vi "initialize Session Data.vi"(0 "OBJ - Session in":refnum<class "FPGA Session.lvclass">, 11 "error in":errorcluster) -> (4 "OBJ - Session out":refnum<class "FPGA Session.lvclass">, 15 "error out":errorcluster)   [LabVIEW 2015, in "FPGA Session.lvclass"]
doc: "OVERRIDE VI\nPlaceholder for decendant sessions to initialize and set their default values"
uses:
  FPGA Session.lvclass
  FPGA Session.lvclass/FPGA Session.ctl
  <vilib>/Utility/error.llb/Error Cluster From Error Code.vi
  <vilib>/rvi/errors/niLvFpgaAdjustHostInterfaceError.vi
  <vilib>/RVI Host/nirviSupport.llb/nirviErrorClusterFromErrorCode.vi
  <vilib>/FPGAPlugInAG/cRIO-9081/niLvFpga_Open_cRIO-9081.vi
  FPGA Ref.ctl
  <vilib>/rvi/interface/nirviMethod/nirviMethod.xnode
  FPGA Bitfiles/NickIO.lvbitx
  <vilib>/rvi/interface/nirviOpenFPGA/nirviOpenFPGA.xnode
  <vilib>/rvi/interface/nirviMethod/StockFPGA_InlinedMethodWaitForSingleIRQ.vi
  <vilib>/FPGAPlugInAG/cRIO-9081/niLvFpga_WaitOnIrq_cRIO-9081.vi
  <vilib>/FPGAPlugInAG/cRIO-9081/niLvFpga_AcknowledgeIrq_cRIO-9081.vi
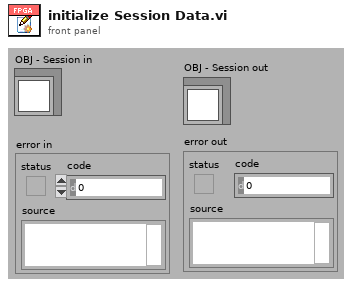
[diagram p1: front panel]
types:
  T1 = typedef "FPGA Ref.ctl" = refnum<k20>
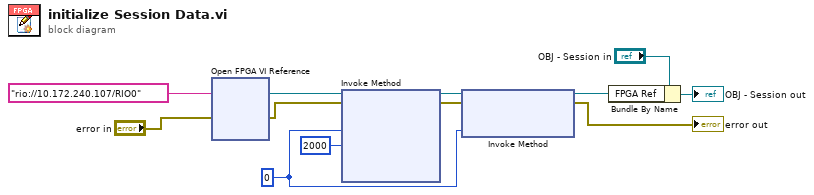
[diagram p0: block diagram]
diagram:
  w5 = 0 ("IRQ Number(s)")
  n1 = xnode "Open FPGA VI Reference"("error in"="error in", "resource name"=tag "rio://10.172.240.107/RIO0") -> ("FPGA VI Reference Out"=w4:T1, "error out"=w3:errorcluster)
  n2 = xnode "Invoke Method"("FPGA VI Reference In"=w4, "error in"=w3, "IRQ Number(s)"=w5, "Timeout (ms)"=2000) -> ("FPGA VI Reference Out"=w7:T1, "error out"=w6:errorcluster)  [unwired: 2 out]
  n3 = xnode "Invoke Method"("FPGA VI Reference In"=w7, "error in"=w6, "IRQ Number(s)"=w5) -> ("FPGA VI Reference Out"=w1:T1, "error out"=→"error out":errorcluster)
  n4 = Bundle By Name(cluster="OBJ - Session in", "FPGA Ref"=w1) -> (→"OBJ - Session out":refnum<class "FPGA Session.lvclass">)
